vi "未命名2.vi"() -> ()   [LabVIEW 2013]
uses:
  <vilib>/Utility/NIReport.llb/NI_report.lvclass
  <vilib>/DAQmx/read.llb/DAQmx Read (Analog Wfm 1Chan NSamp).vi
  <vilib>/addons/_office/excel.llb/Excel Get Data ([str]).vi
  <vilib>/DAQmx/create/channels.llb/DAQmx Create Channel (AI-Voltage-Basic).vi
  <vilib>/DAQmx/configure/timing.llb/DAQmx Timing (Sample Clock).vi
  <vilib>/measure/madcrms.llb/Basic Averaged DC-RMS for 1 Chan.vi
  <vilib>/DAQmx/miscellaneous.llb/DAQmx Fill In Error Info.vi
  <vilib>/addons/_office/NI_ReportGenerationToolkit.lvlib
  <vilib>/measure/NI_MAPro.lvlib
  <vilib>/Utility/NIReport.llb/Excel/NI_Excel.lvclass
panel:
  out "数值":dbl
  out "db值 正确 2":dbl=9.59943087557441
  out "x-y":dbl
  out "db值 正确":dbl=9.59943087557441
  out "error out":errorcluster
  out "CMD":string="MR2;FR98.1MZ;LE66DU;PI10PC;MS90PC;M1;PION"
  in  "VISA资源名称":refnum<visa-resource-name>="GPIB0::2::INSTR"
  out "备注":string="1KHz;98.1MHz;输出66dBu；调制度90+；导频10；立体声主调制"
  out "命令":string="MR2;FR98.1MZ;LE66DU;PI10PC;MS90PC;M1;PION"
  in  "命令列表":u16(ring) items=["FMStereoModulationMain", "FMStereoModulationLeft", "FMStereoModulationRight", "FM信噪比测试", "FM噪限灵敏度90.1MHz", "FM噪限灵敏度106.1MHz", "FM关闭", "FM远程自动停台87.5MHz", "FM远程自动停台98.1MHz", "FM远程自动停台107.9MHz", "FM近程自动停台87.5MHz", "FM近程自动停台98.1MHz", "FM近程自动停台107.9MHz", "FM失真度", "AM远程自动停台603KHz", "AM远程自动停台999KHz", "AM远程自动停台1404KHz", "AM信噪比测试", "AM关闭", "MS关闭", "PI关闭", "恢复默认"]
  in  "Debug":bool=TRUE
  in  "通信协议名称":string
  in  "error in":errorcluster
  out "ConfigPath":string="D:\\导航\\AVN\\config\\FM-AM Signal Generator通信协议.xls"
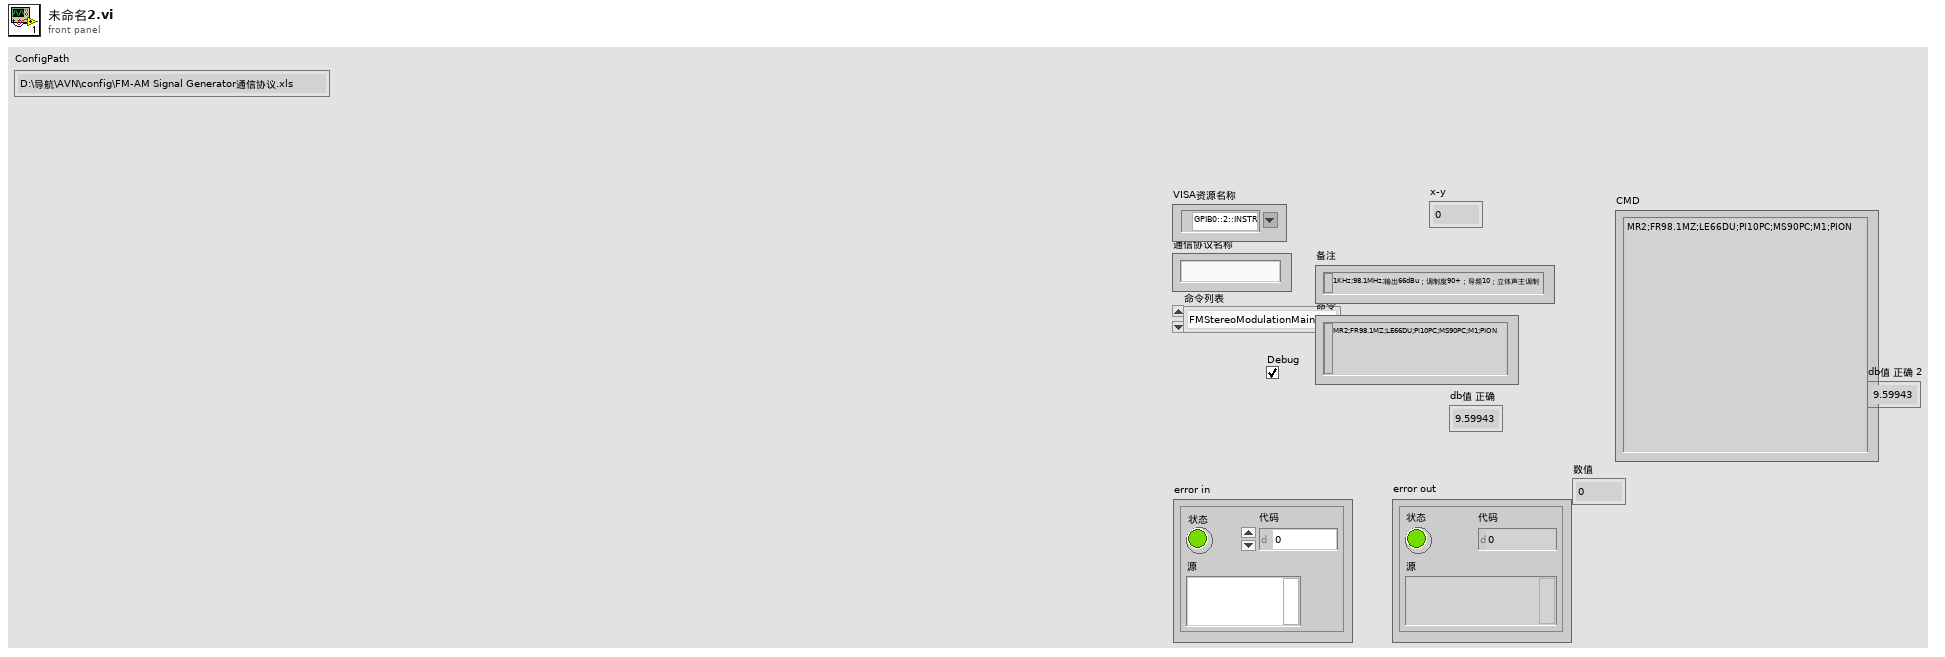
[diagram p1: front panel]
types:
  T1 = enum32{"invalid app kind", "Development System", "Run Time System", "Student Edition", "Embedded LabVIEW", "Evaluation", "Custom"}
  T2 = enum16{"maximized", "minimized", "normal", "no change"}
  T3 = enum16{"Standard Report", "HTML", "Word", "Excel"}
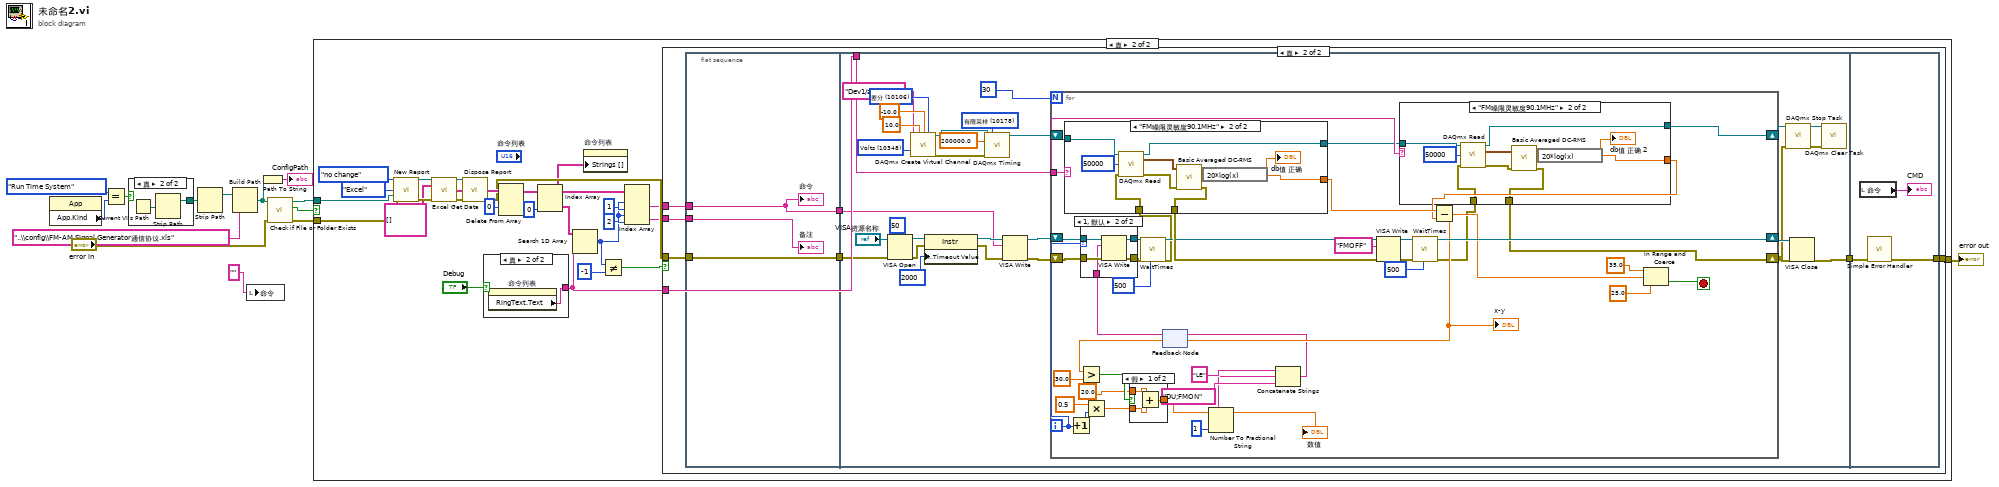
[diagram p0: block diagram]
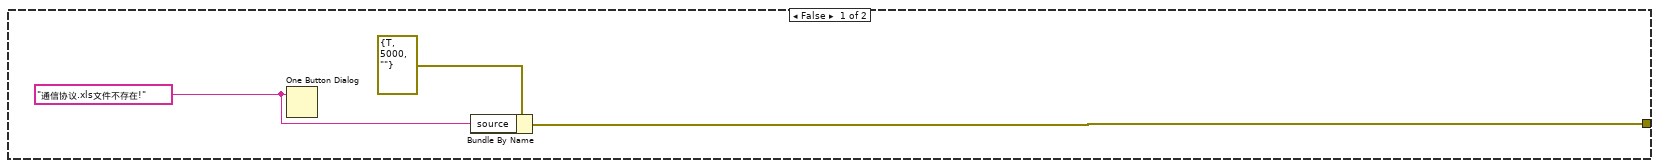
[diagram p2: hidden frame]
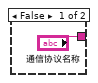
[diagram p3: hidden frame]
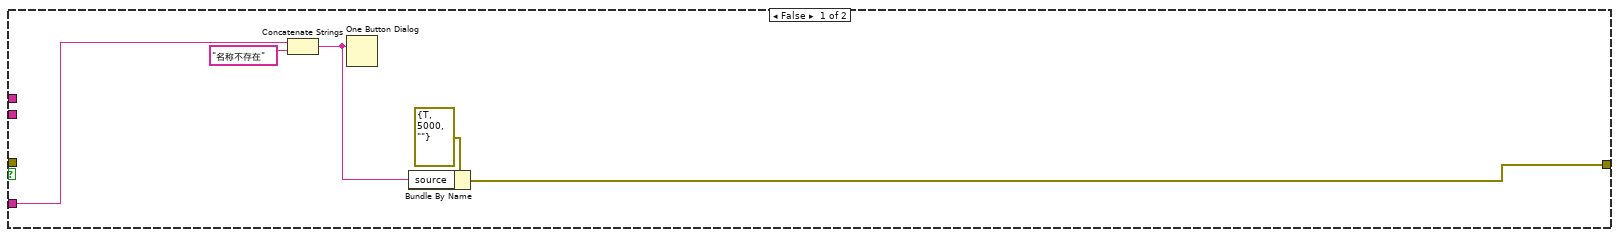
[diagram p4: hidden frame]
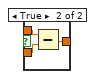
[diagram p7: hidden frame]
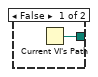
[diagram p9: hidden frame]
diagram:
  n1 = property class="App"() -> ("App.Kind"=w12:T1)  [unwired: 2 in, 2 out]
  n2 = Equal?(x=T1."Run Time System" ("y"), y=w12) -> (x = y?=w14:bool)
  n3 = case shown="真" w14 {
    tunnel: [w15 w17] -> w13
    frame False {
      n4 = Current VI's Path() -> (path=w15:path)
    }
    frame True {
      n5 = Current VI's Path() -> (path=w16:path)
      n6 = Strip Path(path=w16) -> (stripped path=w17:path)  [unwired: 1 out]
    }
  }
  n7 = Strip Path(path=w13) -> (stripped path=w6:path)  [unwired: 1 out]
  n8 = Build Path(base path=w6, name or relative path="..\\config\\FM-AM Signal Generator通信协议.xls" ("连接的字符串")) -> (appended path=w8:path)
  n9 = local write "命令"("" ("响应")) -> ()
  n10 = Path To String(path=w8) -> (string=→"ConfigPath":string)
  n11 = call <vilib>:"Check if File or Folder Exists.vi"("error in (no error)"="error in", "path"=w8) -> ("error out"=w2:errorcluster, "file or folder exists?"=w5:bool, "dup path"=w4:path)  [unwired: 7 out]
  n12 = case shown="真" w5 {
    tunnel: w4 -> [_ w32]
    tunnel: w2 -> [_ w27]
    tunnel: [w19 w26] -> w1
    frame False {
      w18 = "通信协议.xls文件不存在!" ("消息")
      n13 = One Button Dialog(message=w18) -> ()  [unwired: 1 in, 1 out]
      n14 = Bundle By Name(cluster=errorcluster {"status"=TRUE, "code"=5000, "source"=""} ("error in 1 (no error)"), "source"=w18) -> (w19:errorcluster)
    }
    frame True {
      n15 = call <vilib>:"New Report.vi"("window state (normal)"=T2."no change", "report type"=T3."Excel", "template (empty)"=w32, "error in (no error)"=w27) -> ("report out"=w40:refnum<class "NI_report.lvclass">, "error out"=w41:errorcluster)  [unwired: 2 in, 8 out]
      n16 = call-poly <vilib>:"Excel Get Data.vi"("report in"=w40, "data type"=string[][] [], "error in (no error)"=w41) -> ("report out"=w37:refnum<class "NI_report.lvclass">, "data"=w42:string[][], "error out"=w36:errorcluster)  [unwired: 10 in]
      n17 = call-dynamic "Dispose Report.vi"("report in"=w37, "error in (no error)"=w36) -> ("error out"=w28:errorcluster)  [unwired: 3 in, 10 out]
      n18 = case shown="真" "Debug" {
        tunnel: ["通信协议名称" w47] -> w21
        frame False {
        }
        frame True {
          n19 = property on="命令列表" class="Ring (严格)"() -> ("RingText.Text"=w47:string)  [unwired: 2 in, 2 out]
        }
      }
      n20 = Delete From Array(array=w42, index (row)=0 ("索引 (行)")) -> (array with subset deleted=w35:string[][])  [unwired: 2 in, 1 out]
      n21 = Index Array(array=w35, index (col)=0 ("禁用的索引 (列)")) -> (element=w25:string[])  [unwired: 1 in]
      n22 = Search 1D Array(1D array=w25, element=w21) -> (index of element=w31:i32)  [unwired: 1 in]
      n23 = property on="命令列表" class="Ring (严格)"("Strings []"=w25) -> ()  [unwired: 2 in, 2 out]
      n24 = Not Equal?(x=w31, y=-1) -> (x != y?=w29:bool)
      n25 = Index Array(array=w35, index (row) #1=w31, index (col) #1=1 ("索引 (列)"), index (row) #2=w31, index (col) #2=2 ("索引 (列)")) -> (element #1=w23:string, element #2=w22:string)
      n26 = case shown="真" w29 {
        tunnel: w23 -> [_ w59]
        tunnel: w28 -> [_ w58]
        tunnel: [w49 w56] -> w26
        tunnel: w22 -> [_ w54]
        tunnel: w21 -> [w48 w53]
        frame False {
          n27 = Concatenate Strings(w48, "名称不存在" ("消息")) -> (w50:string)
          n28 = One Button Dialog(message=w50) -> ()  [unwired: 1 in, 1 out]
          n29 = Bundle By Name(cluster=errorcluster {"status"=TRUE, "code"=5000, "source"=""} ("error in 1 (no error)"), "source"=w50) -> (w49:errorcluster)
        }
        frame True {
          n30 = flat-sequence {
            tunnel: [w61] -> w60
            tunnel: w59 -> [w61]
            tunnel: w58 -> [w63]
            tunnel: [w63] -> w57
            tunnel: w54 -> [w62]
            tunnel: w60 -> [w78]
            tunnel: w57 -> [w86]
            tunnel: [w92] -> w55
            tunnel: w53 -> [w85]
            tunnel: [w165] -> w56
            tunnel: w55 -> [w166]
            frame #0 {
              "备注" <- w62
              "命令" <- w61
            }
            frame #1 {
              w72 = 10178 items=["有限采样"=10178, "连续采样"=10123, "硬件定时单点"=12522] ("sample mode")
              w75 = 10106 items=["默认"=-1, "RSE"=10083, "NRSE"=10078, "差分"=10106, "伪差分"=12529] ("input terminal configuration")
              w76 = 10348 items=["Volts"=10348, "From Custom Scale"=10065] ("units")
              n31 = VISA Open(timeout (0)=u32 50 ("VISA Open timeout"), error in (no error)=w86, VISA resource name="VISA资源名称") -> (VISA resource name=w89:refnum<visa-resource-name>, error out=w88:errorcluster)  [unwired: 2 in]
              n32 = call-poly <vilib>:"DAQmx Create Virtual Channel.vi"("maximum value"=10.0, "minimum value"=-10.0, "input terminal configuration"=w75, "physical channels"=tag "Dev1/ai0", "units"=w76) -> ("task out"=w70:refnum<k21>, "error out"=w71:errorcluster)  [unwired: 9 in]
              n33 = property class="Instr"(reference=w89, error in=w88, "General Settings:Timeout Value"=u32 2000 ("Timeout")) -> (reference out=w80:refnum<visa-resource-name>, error out=w82:errorcluster)
              n34 = call-poly <vilib>:"DAQmx Timing.vi"("task/channels in"=w70, "sample mode"=w72, "rate"=200000.0, "error in"=w71) -> ("task out"=w64:refnum<k21>)  [unwired: 3 in, 8 out]
              n35 = VISA Write(VISA resource name=w80, write buffer=w78, error in (no error)=w82) -> (VISA resource name out=w79:refnum<visa-resource-name>, error out=w81:errorcluster)  [unwired: 1 out]
              n36 = for {
                N: 30 -> [_]
                tunnel: w85 -> [w115]
                shift-right: [w108] -> w68
                shift-left: w81 -> [w114]
                shift-right: [w126] -> w84
                shift-left: w79 -> [w113]
                shift-right: [w93] -> w67
                shift-left: w64 -> [w95]
                i -> [w99]
                stop <- w129 stop-if-true
                n37 = Increment(x=w99) -> (x+1=w98:i32)
                n38 = Multiply(x=0.5, y=w98) -> (x*y=w117:dbl)
                n39 = feedback #1() -> (w106:string)  [unwired: 1 in]
                n40 = case shown="1, 默认" w99 {
                  tunnel: w114 -> [w130 w136]
                  tunnel: w113 -> [w131 w135]
                  tunnel: [w131 w134] -> w112
                  tunnel: [w130 w133] -> w102
                  tunnel: w106 -> [_ w132]
                  frame 0 {
                  }
                  frame 1, Default {
                    n41 = VISA Write(VISA resource name=w135, write buffer=w132, error in (no error)=w136) -> (VISA resource name out=w134:refnum<visa-resource-name>, error out=w133:errorcluster)  [unwired: 1 out]
                  }
                }
                n42 = call "WaitTimes.vi"("WaitTimes"=u32 500, "error in (no error)"=w102) -> ("error out"=w101:errorcluster)  [unwired: 9 in]
                n43 = case shown="\"FM噪限灵敏度90.1MHz\"" w115 {
                  tunnel: w101 -> [w155 w158]
                  tunnel: [w155 w159] -> w116
                  tunnel: [_ w163] -> w111
                  tunnel: w95 -> [w154 w157]
                  tunnel: [w154 w160] -> w94
                  frame "假", Default {
                  }
                  frame "FM噪限灵敏度90.1MHz" {
                    n44 = call-poly <vilib>:"DAQmx Read.vi"("task/channels in"=w157, "number of samples per channel"=50000, "error in"=w158) -> ("task out"=w160:refnum<k21>, "data"=w156:waveform(dbl), "error out"=w161:errorcluster)  [unwired: 10 in]
                    n45 = call-poly <vilib>:"Basic Averaged DC-RMS.vi"("error in (no error)"=w161, "signal in"=w156) -> ("error out"=w159:errorcluster, "RMS value"=w164:dbl)  [unwired: 6 in, 2 out]
                    n46 = expression code="20*log(x)"(w164) -> (w163:dbl)
                    "db值 正确" <- w163
                  }
                }
                n47 = VISA Write(VISA resource name=w112, write buffer="FMOFF" ("写入缓冲区"), error in (no error)=w116) -> (VISA resource name out=w126:refnum<visa-resource-name>, error out=w105:errorcluster)  [unwired: 1 out]
                n48 = call "WaitTimes.vi"("WaitTimes"=u32 500, "error in (no error)"=w105) -> ("error out"=w104:errorcluster)  [unwired: 9 in]
                n49 = case shown="\"FM噪限灵敏度90.1MHz\"" w115 {
                  tunnel: w104 -> [w138 w142]
                  tunnel: [w138 w141] -> w108
                  tunnel: [_ w146] -> w110
                  tunnel: w94 -> [w137 w144]
                  tunnel: [w137 w140] -> w93
                  frame "假", Default {
                  }
                  frame "FM噪限灵敏度90.1MHz" {
                    n50 = call-poly <vilib>:"DAQmx Read.vi"("task/channels in"=w144, "number of samples per channel"=50000, "error in"=w142) -> ("task out"=w140:refnum<k21>, "data"=w139:waveform(dbl), "error out"=w143:errorcluster)  [unwired: 10 in]
                    n51 = call-poly <vilib>:"Basic Averaged DC-RMS.vi"("error in (no error)"=w143, "signal in"=w139) -> ("error out"=w141:errorcluster, "RMS value"=w147:dbl)  [unwired: 6 in, 2 out]
                    n52 = expression code="20*log(x)"(w147) -> (w146:dbl)
                    "db值 正确 2" <- w146
                  }
                }
                n53 = Subtract(x=w111, y=w110) -> (x-y=w125:dbl)
                "x-y" <- w125
                n54 = Greater?(x=w125, y=30.0) -> (0:w119:bool)
                n55 = case shown="假" w119 {
                  tunnel: 20.0 ("x") -> [w149 w153]
                  tunnel: w117 -> [w150 w152]
                  tunnel: [w148 w151] -> w97
                  frame False {
                    n56 = Add(x=w149, y=w150) -> (x+y=w148:dbl)
                  }
                  frame True {
                    n57 = Subtract(x=w153, y=w152) -> (x-y=w151:dbl)
                  }
                }
                "数值" <- w97
                n58 = Number To Fractional String(number=w97, precision (6)=i16 1 ("精度(6)")) -> (F-format string=w120:string)  [unwired: 2 in]
                n59 = Concatenate Strings("LE" ("Mode"), w120, "DU;FMON" ("Mode")) -> (w107:string)
                n60 = feedback-in #1(w107) -> ()
                n61 = In Range and Coerce(upper limit=35.0 ("上限"), x=w125, lower limit=25.0 ("下限")) -> (In Range?=w129:bool)  [unwired: 1 out]
              }
              n62 = call <vilib>:"DAQmx Stop Task.vi"("task/channels in"=w67, "error in"=w68) -> ("task out"=w66:refnum<k21>, "error out"=w69:errorcluster)  [unwired: 12 in]
              n63 = VISA Close(VISA resource name=w84, error in (no error)=w68) -> (error out=w92:errorcluster)
              n64 = call <vilib>:"DAQmx Clear Task.vi"("task in"=w66, "error in"=w69) -> ()  [unwired: 13 in, 1 out]
            }
            frame #2 {
              n65 = local read "命令"() -> (→"CMD":string)
              n66 = call <vilib>:"Simple Error Handler.vi"("error in (no error)"=w166) -> ("error out"=w165:errorcluster)  [unwired: 4 in, 4 out]
            }
          }
        }
      }
    }
  }
  "error out" <- w1
